vi "DSF.Transceiver.UDP.Errors Info.vi"(11 "Error":T1) -> (2 "description":string, 3 "code":i32)   [LabVIEW 2017, in "DSF.Transceiver.UDP.lvlib" / "DSF.Transceiver.UDP.lvclass"]
uses:
  DSF.Transceiver.UDP.lvclass
  DSF.Transceiver.UDP.Errors.ctl
  DSF.Transceiver.UDP.Constants.Base Error Code.vi
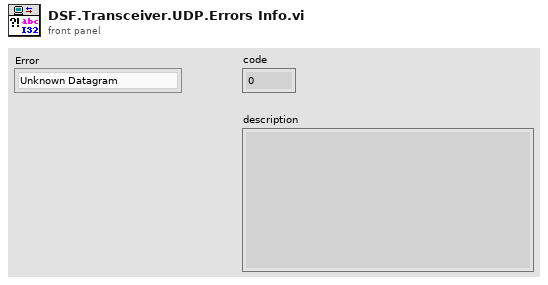
[diagram p1: front panel]
types:
  T1 = typedef "DSF.Transceiver.UDP.lvlib/DSF.Transceiver.UDP.lvclass/DSF.Transceiver.UDP.Errors.ctl" = enum16{"Unknown Datagram", "Size Mismatch"}
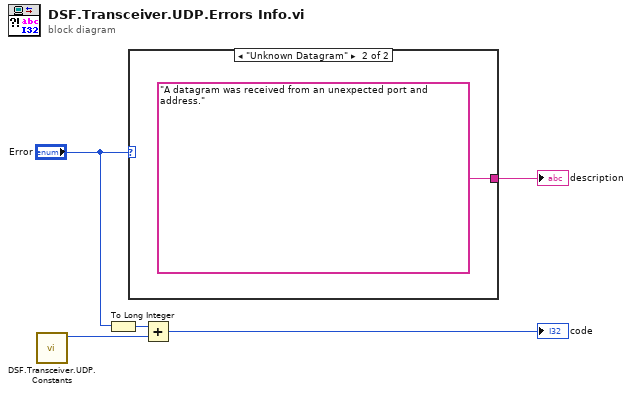
[diagram p0: block diagram]
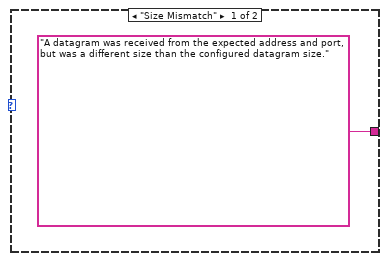
[diagram p2: hidden frame]
diagram:
  n1 = call-poly "DSF.Transceiver.UDP.Constants.vi"() -> ("base error code"=w5:i32)  [unwired: 11 in]
  n2 = To Long Integer(number="Error") -> (32bit integer=w4:i32)
  n3 = case shown="\"Unknown Datagram\"" "Error" {
    tunnel: ["A datagram was received from the expected address and port, but was a different size than the configured datagram size." "A datagram was received from an unexpected port and address."] -> w1
    frame "Size Mismatch" {
    }
    frame "Unknown Datagram" {
    }
  }
  "description" <- w1
  n4 = Add(x=w4, y=w5) -> (x+y=→"code":i32)
